vi "DSF.Transceiver.UDP.Get Buffer.vi"(11 "DSF.Transceiver.UDP in":refnum<class "DSF.Transceiver.UDP.lvclass">) -> (2 "buffer":u8[](array[numeric]), 3 "DSF.Transceiver.UDP out":refnum<class "DSF.Transceiver.UDP.lvclass">)   [LabVIEW 2017, in "DSF.Transceiver.UDP.lvlib" / "DSF.Transceiver.UDP.lvclass"]
uses:
  DSF.Transceiver.UDP.lvclass
  DSF.Transceiver.UDP.lvclass/DSF.Transceiver.UDP.ctl
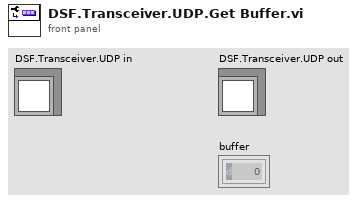
[diagram p1: front panel]
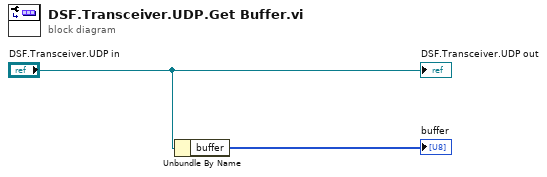
[diagram p0: block diagram]
diagram:
  n1 = Unbundle By Name("DSF.Transceiver.UDP in") -> ("buffer"=→"buffer":u8[])
  "DSF.Transceiver.UDP out" <- "DSF.Transceiver.UDP in"
